vi "GetDevices.vi"(11 "Base URL":string) -> (0 "error out":errorcluster, 1 "Types":string[](array[string]), 2 "Names":string[](array[string]), 3 "Devices":T1[](array[typedef]))   [LabVIEW 2026]
uses:
  SensorCluster.ctl
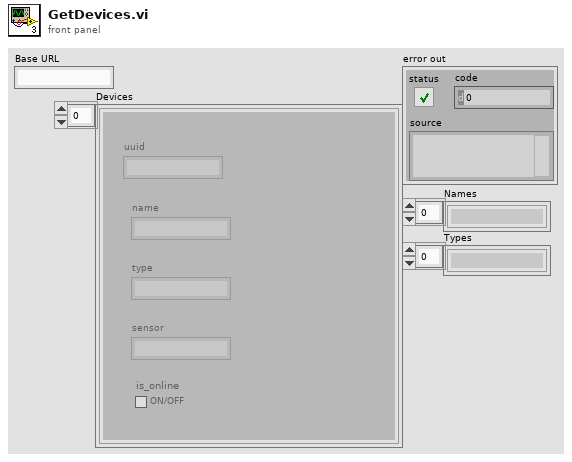
[diagram p1: front panel]
types:
  T1 = typedef "SensorCluster.ctl" = cluster{"uuid":string, "name":string, "type":string, "sensor":string, "is_online":bool}
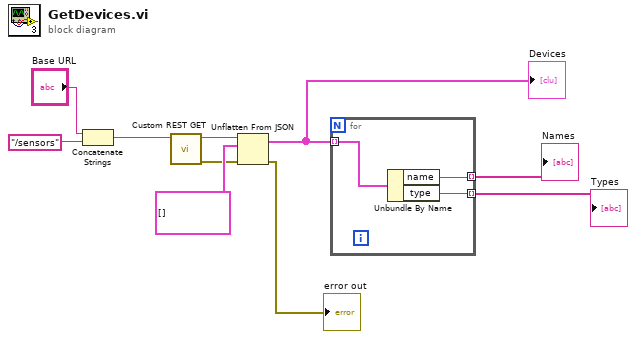
[diagram p0: block diagram]
diagram:
  n1 = Concatenate Strings("Base URL", "/sensors" ("string")) -> (w9:string)
  n2 = call "Custom REST GET.vi"("Base URL"=w9) -> ("Error out"=w3:errorcluster, "body"=w10:string)  [unwired: 9 in]
  n3 = Unflatten From JSON(JSON string=w10, type and defaults=T1[] [], error in (no error)=w3) -> (value=w1:T1[], error out=→"error out":errorcluster)  [unwired: 4 in]
  "Devices" <- w1
  n4 = for {
    tunnel: w1 -> [w13] mode=indexing
    tunnel: [w12] -> w7 mode=indexing
    tunnel: [w11] -> w6 mode=indexing
    n5 = Unbundle By Name(w13) -> ("name"=w12:string, "type"=w11:string)
  }
  "Names" <- w7
  "Types" <- w6
